vi "Run FGV Tests for VI Refnum.vi"(2 "DELETE VI Reference":refnum<vi>, 3 "GET VI Reference":refnum<vi>, 4 "PUT VI Reference":refnum<vi>) -> (0 "Reason":string, 1 "Success":bool)   [LabVIEW 2013]
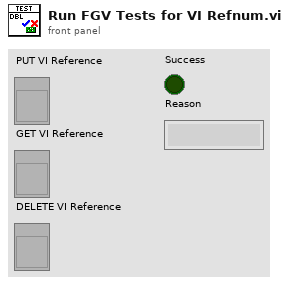
[diagram p1: front panel]
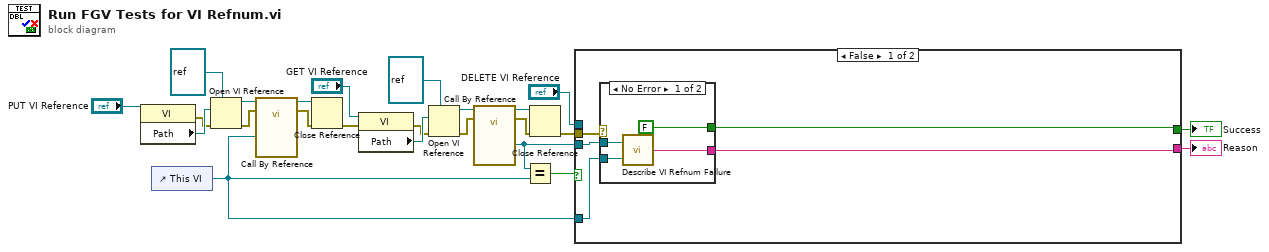
[diagram p0: block diagram]
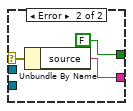
[diagram p2: hidden frame]
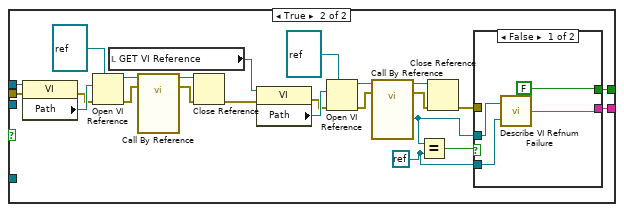
[diagram p3: hidden frame]
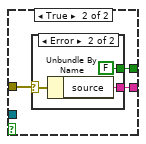
[diagram p4: hidden frame]
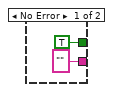
[diagram p5: hidden frame]
diagram:
  n1 = property class="VI"(reference="PUT VI Reference") -> (error out=w4:errorcluster, "Path"=w15:path)  [unwired: 1 in, 1 out]
  n2 = control-ref of="This VI"() -> (w1:refnum<vi>)
  n3 = Open VI Reference(type specifier VI Refnum (for type only)=refnum<vi> refnum, vi path=w15, error in (no error)=w4) -> (vi reference=w14:refnum<vi>, error out=w13:errorcluster)  [unwired: 3 in]
  n4 = call-by-ref "?"(reference=w14, error in=w13, "Experimental Data Save VI Reference"=w1) -> (reference out=w12:refnum<vi>, error out=w11:errorcluster)
  n5 = Close Reference(reference=w12, error in (no error)=w11) -> (error out=w9:errorcluster)
  n6 = property class="VI"(reference="GET VI Reference", error in=w9) -> (error out=w5:errorcluster, "Path"=w20:path)  [unwired: 1 out]
  n7 = Open VI Reference(type specifier VI Refnum (for type only)=refnum<vi> refnum, vi path=w20, error in (no error)=w5) -> (vi reference=w21:refnum<vi>, error out=w22:errorcluster)  [unwired: 3 in]
  n8 = call-by-ref "?"(reference=w21, error in=w22) -> (reference out=w23:refnum<vi>, error out=w24:errorcluster, "Experimental VI Reference"=w6:refnum<vi>)
  n9 = Equal?(x=w6, y=w1) -> (x = y?=w7:bool)
  n10 = Close Reference(reference=w23, error in (no error)=w24) -> (error out=w8:errorcluster)
  n11 = case shown="False" w7 {
    tunnel: "DELETE VI Reference" -> [_ w54]
    tunnel: w8 -> [w25 w53]
    tunnel: w1 -> [w28 _]
    tunnel: w6 -> [w29 _]
    tunnel: [w27 w39] -> w3
    tunnel: [w26 w38] -> w2
    frame False {
      n12 = case shown="No Error" w25 {
        selector: w25 -> [_ w36]
        tunnel: w29 -> [w33 _]
        tunnel: w28 -> [w32 _]
        tunnel: [FALSE FALSE] -> w27
        tunnel: [w30 w34] -> w26
        frame No Error {
          n13 = call "Describe VI Refnum Failure.vi"("Expected"=w32, "Got"=w33) -> ("Failure Description"=w30:string)
        }
        frame Error {
          n14 = Unbundle By Name(w36) -> ("source"=w34:string)
        }
      }
    }
    frame True {
      w37 = refnum<k0> refnum
      n15 = property class="VI"(reference=w54, error in=w53) -> (error out=w43:errorcluster, "Path"=w56:path)  [unwired: 1 out]
      n16 = Open VI Reference(type specifier VI Refnum (for type only)=refnum<vi> refnum, vi path=w56, error in (no error)=w43) -> (vi reference=w57:refnum<vi>, error out=w58:errorcluster)  [unwired: 3 in]
      n17 = local read "GET VI Reference"() -> (w41:refnum<vi>)
      n18 = call-by-ref "?"(reference=w57, error in=w58) -> (reference out=w59:refnum<vi>, error out=w60:errorcluster)  [unwired: 1 in]
      n19 = Close Reference(reference=w59, error in (no error)=w60) -> (error out=w46:errorcluster)
      n20 = property class="VI"(reference=w41, error in=w46) -> (error out=w44:errorcluster, "Path"=w48:path)  [unwired: 1 out]
      n21 = Open VI Reference(type specifier VI Refnum (for type only)=refnum<vi> refnum, vi path=w48, error in (no error)=w44) -> (vi reference=w49:refnum<vi>, error out=w50:errorcluster)  [unwired: 3 in]
      n22 = call-by-ref "?"(reference=w49, error in=w50) -> (reference out=w51:refnum<vi>, error out=w52:errorcluster, "Experimental VI Reference"=w40:refnum<vi>)
      n23 = Equal?(x=w40, y=w37) -> (x = y?=w45:bool)
      n24 = Close Reference(reference=w51, error in (no error)=w52) -> (error out=w42:errorcluster)
      n25 = case shown="False" w45 {
        tunnel: w42 -> [_ w67]
        tunnel: w40 -> [w64 _]
        tunnel: w37 -> [w63 _]
        tunnel: [FALSE w66] -> w39
        tunnel: [w61 w65] -> w38
        frame False {
          n26 = call "Describe VI Refnum Failure.vi"("Expected"=w63, "Got"=w64) -> ("Failure Description"=w61:string)
        }
        frame True {
          n27 = case shown="Error" w67 {
            selector: w67 -> [_ w72]
            tunnel: [TRUE FALSE] -> w66
            tunnel: ["" ("source") w70] -> w65
            frame No Error {
            }
            frame Error {
              n28 = Unbundle By Name(w72) -> ("source"=w70:string)
            }
          }
        }
      }
    }
  }
  "Success" <- w3
  "Reason" <- w2
